vi "Send test DATA.vi"(7 "isInt?":bool, 8 "errin":errorcluster, 9 "Value":dbl, 10 "SN":string, 11 "test":string="InsuP") -> (0 "error out":errorcluster)   [LabVIEW 2020]
uses:
  <userlib>/Sylvain.lib/DATA_INSERT.vi
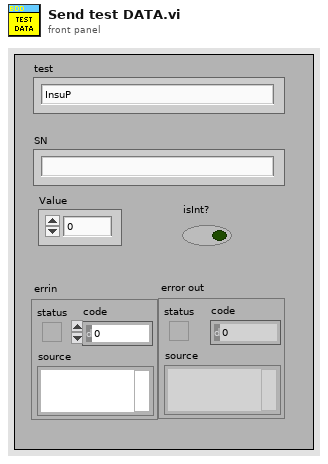
[diagram p1: front panel]
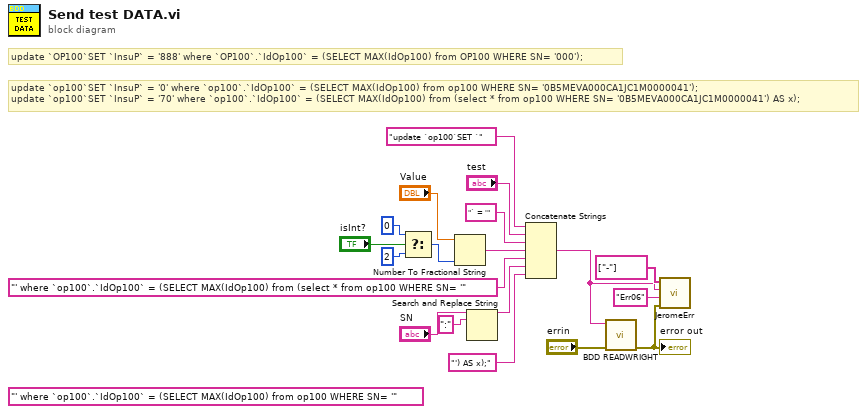
[diagram p0: block diagram]
diagram:
  (unwired) "' where `op100`.`IdOp100` = (SELECT MAX(IdOp100) from op100 WHERE SN= '" ("chaîne")
  # "update `op100`SET `InsuP` = '0' where `op100`.`IdOp100` = (SELECT MAX(IdOp100) from op100 WHERE SN= '0B5MEVA000CA1JC1M0000041');\nupdate `op100`SET `InsuP` = '70' where `op100`.`IdOp100` = (SELECT MAX(IdOp100) from (select * from op100 WHERE SN= '0B5MEVA000CA1JC1M0000041') AS x);"
  # "update `OP100`SET `InsuP` = '888' where `OP100`.`IdOp100` = (SELECT MAX(IdOp100) from OP100 WHERE SN= '000');"
  n1 = Select ("Sélectionner")(t=i16 0 ("cas vrai"), s="isInt?", f=i16 2 ("précision (6)")) -> (s? t:f=w6:i16)
  n2 = Number To Fractional String ("Nombre en chaîne fractionnaire")(number="Value", precision (6)=w6) -> (F-format string=w15:string)  [unwired: 2 in]
  n3 = Search and Replace String ("Rechercher et remplacer une chaîne")(input string="SN", search string=":" ("chaîne recherchée")) -> (result string=w12:string)  [unwired: 6 in, 3 out]
  n4 = Concatenate Strings("update `op100`SET `" ("chaîne"), "test", "` = '" ("chaîne"), w15, "' where `op100`.`IdOp100` = (SELECT MAX(IdOp100) from (select * from op100 WHERE SN= '" ("chaîne"), w12, "') AS x);" ("chaîne")) -> (w2:string)
  n5 = call "BDD READWRIGHT.vi"("errin"="errin", "INSERT"=w2) -> ("errout"=w1:errorcluster)  [unwired: 9 in]
  "error out" <- w1
  n6 = call "JeromeErr.vi"("Errin"=w1, "CodeERR"="Err06", "RequetteSQL"=w2, "RetourSQL"=string[] ["-"]) -> ()  [unwired: 7 in, 1 out]
